vi "send_command_to_address.vi"(6 "address_group":u16 format="%x", 7 "addressing_type":T1="4", 8 "error in (no error)":errorcluster, 9 "command_data":u32 format="%x", 10 "command":u32, 11 "device_handle":i32) -> (0 "error out":errorcluster, 1 "failstring":string, 2 "ok":bool, 3 "response_command":i32)   [LabVIEW 2014, in "Dali_usb.lvlib"]
uses:
  Dali_usb.lvlib
  Controls/Addressing_type.ctl
  dll/DaliBusAccess.dll
panel:
  # "int32_t SendBusData(\nint32_t hDeviceHandle, \nuint32_t dwBusCommand, \nuint32_t dwBusData, \nuint32_t dwFlags, \nuint16_t wBusAddress, \nuint32_t dwAdditionalData, \nuint32_t dwAdditionalAddress);"
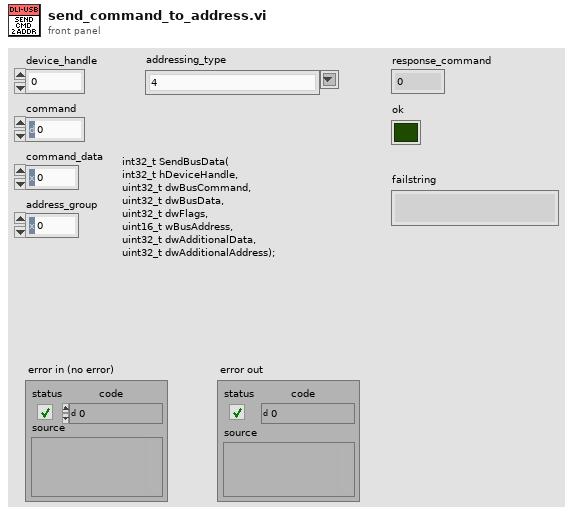
[diagram p1: front panel]
types:
  T1 = typedef "Dali_usb.lvlib/Addressing_type.ctl" = string
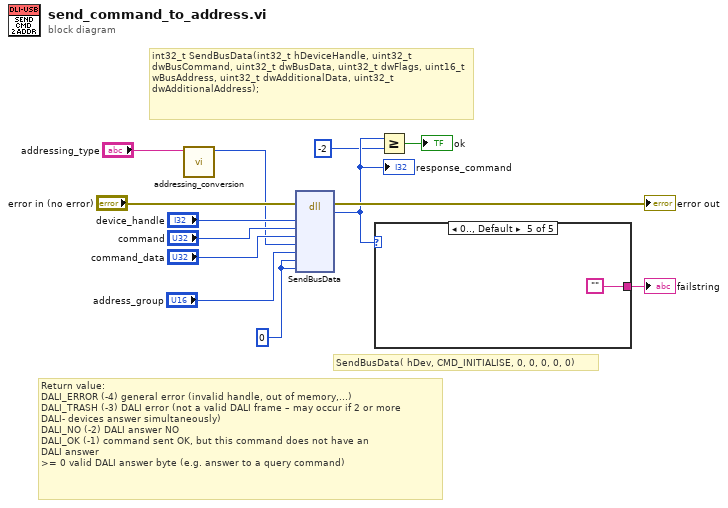
[diagram p0: block diagram]
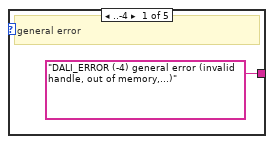
[diagram p2: hidden frame]
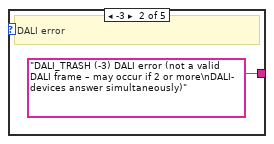
[diagram p3: hidden frame]
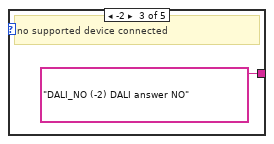
[diagram p4: hidden frame]
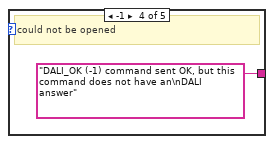
[diagram p5: hidden frame]
diagram:
  w10 = u32 0 ("dwAdditionalData")
  # "SendBusData( hDev, CMD_INITIALISE, 0, 0, 0, 0, 0)"
  # "int32_t SendBusData(int32_t hDeviceHandle, uint32_t dwBusCommand, uint32_t dwBusData, uint32_t dwFlags, uint16_t wBusAddress, uint32_t dwAdditionalData, uint32_t dwAdditionalAddress);"
  # "Return value: \nDALI_ERROR (-4) general error (invalid handle, out of memory,...)\nDALI_TRASH (-3) DALI error (not a valid DALI frame – may occur if 2 or more\nDALI- devices answer simultaneously)\nDALI_NO (-2) DALI answer NO\nDALI_OK (-1) command sent OK, but this command does not have an\nDALI answer\n>= 0 valid DALI answer byte (e.g. answer to a query command)"
  n1 = call "addressing_conversion.vi"("addressing_type"="addressing_type") -> ("addressing_number"=w1:u32)  [unwired: 10 in]
  n2 = dll-call lib="C:/LTS/app-tde-luminaires/SourceCode/Instruments/Driver_interaction/Dali_usb/Vendor/dll/DaliBusAccess.dll" fn="SendBusData"(error in="error in (no error)", "hDeviceHandle"="device_handle", "dwBusCommand"="command", "dwBusData"="command_data", "dwFlags"=w1, "wBusAddress"="address_group", "dwAdditionalData"=w10, "dwAdditionalAddress"=w10) -> (error out=→"error out":errorcluster, "return type"=w4:i32)  [unwired: 9 in, 1 out]
  "response_command" <- w4
  n3 = case shown="0.., Default" w4 {
    tunnel: ["DALI_ERROR (-4) general error (invalid handle, out of memory,...)" "DALI_TRASH (-3) DALI error (not a valid DALI frame – may occur if 2 or more\nDALI- devices answer simultaneously)" "DALI_NO (-2) DALI answer NO" "DALI_OK (-1) command sent OK, but this command does not have an\nDALI answer" ""] -> w6
    frame ..-4 {
      # "general error"
    }
    frame -3 {
      # "DALI error"
    }
    frame -2 {
      # "no supported device connected"
    }
    frame -1 {
      # "could not be opened"
    }
    frame 0.., Default {
    }
  }
  "failstring" <- w6
  n4 = Greater Or Equal?(x=w4, y=-2) -> (x >= y?=→"ok":bool)
